vi "No Trip Tests at 120mA.vi"(3 "error in":errorcluster) -> (10 "error out":errorcluster)   [LabVIEW 2015]
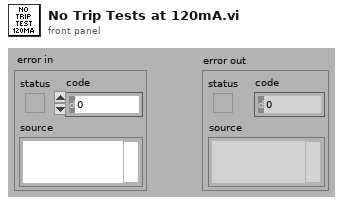
[diagram p1: front panel]
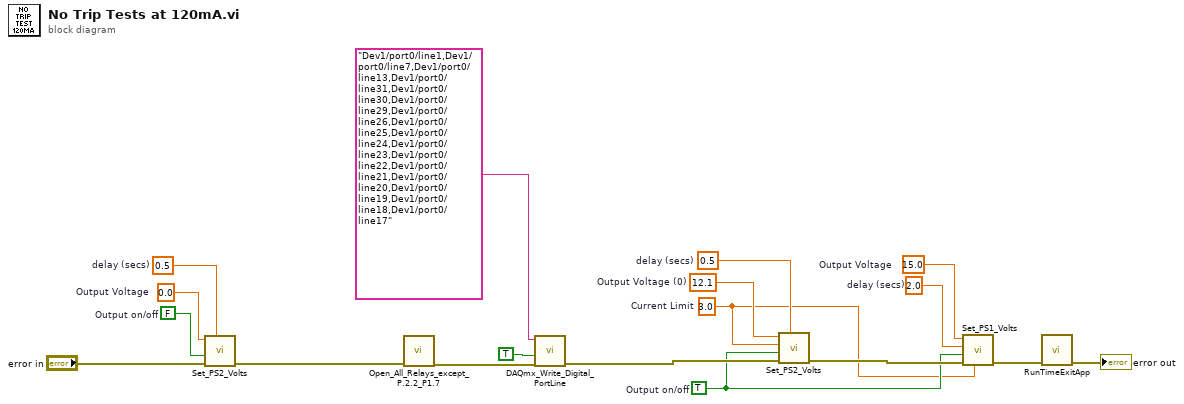
[diagram p0: block diagram]
diagram:
  w2 = 0.5  # delay (secs)
  w3 = 15.0  # Output Voltage
  w1 = 3.0  # Current Limit
  w11 = 0.0  # Output Voltage
  w12 = 0.5  # delay (secs)
  w13 = FALSE  # Output on/off
  w4 = TRUE  # Output on/off
  w5 = 2.0  # delay (secs)
  w6 = 12.1  # Output Voltage (0)
  n1 = call "Set_PS2_Volts.vi"("delay (secs)"=w12, "error in"="error in", "Output on/off"=w13, "Output Voltage"=w11) -> ("error out"=w14:errorcluster)  [unwired: 5 in, 2 out]
  n2 = call "Open_All_Relays_except_P.2.2_P1.7.vi"("error in"=w14) -> ("error out"=w15:errorcluster)  [unwired: 8 in]
  n3 = call "DAQmx_Write_Digital_PortLine.vi"("Device/Ports/Lines"="Dev1/port0/line1,Dev1/port0/line7,Dev1/port0/line13,Dev1/port0/line31,Dev1/port0/line30,Dev1/port0/line29,Dev1/port0/line26,Dev1/port0/line25,Dev1/port0/line24,Dev1/port0/line23,Dev1/port0/line22,Dev1/port0/line21,Dev1/port0/line20,Dev1/port0/line19,Dev1/port0/line18,Dev1/port0/line17", "Boolean"=TRUE, "error in"=w15) -> ("error out"=w17:errorcluster)  [unwired: 6 in, 1 out]
  n4 = call "Set_PS2_Volts.vi"("delay (secs)"=w2, "error in"=w17, "Output on/off"=w4, "Current Limit"=w1, "Output Voltage"=w6) -> ("error out"=w8:errorcluster)  [unwired: 4 in, 2 out]
  n5 = call "Set_PS1_Volts.vi"("Current Limit (0)"=w1, "error in"=w8, "Output on/off"=w4, "delay (secs)"=w5, "Output Voltage"=w3) -> ("error out"=w7:errorcluster)  [unwired: 4 in, 2 out]
  n6 = call "RunTimeExitApp.vi"("error in (no error)"=w7) -> ("error out"=→"error out":errorcluster)  [unwired: 10 in]
